vi "Configure TV Trig HDTV Format.vi"(8 "error in (no error)":errorcluster {"code" format="%.0x"}, 10 "HDTV Format (1080I50)":i32(slide), 11 "VISA Resource Name":refnum<visa-resource-name>) -> (0 "error out":errorcluster {"code" format="%.0x"}, 3 "VISA Resource Name Out":refnum<visa-resource-name>)   [LabVIEW 2010, in "Tektronix TDS 3000 Series.lvlib"]
doc: "This VI configures the HDTV settings for the HDTV TV triggering.\n\nNotes:\n\n(1) This VI is effective only if TV Trigger Signal Format in Configure TV Trigger Source is selected as HDTV"
uses:
  <instrlib>/Tektronix TDS 3000 Series/Tektronix TDS 3000 Series.lvlib
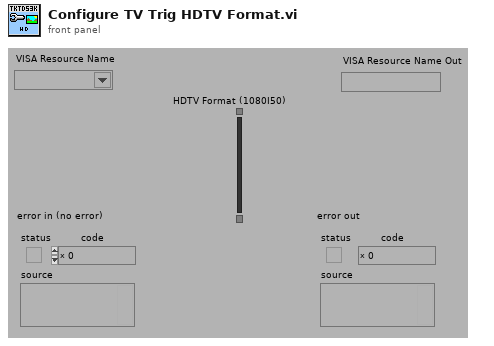
[diagram p1: front panel]
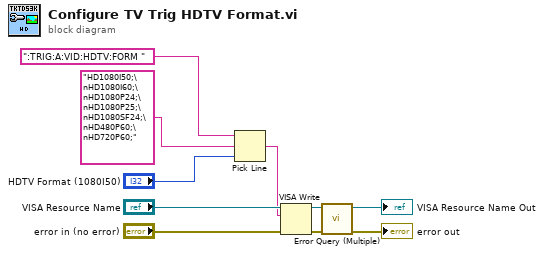
[diagram p0: block diagram]
diagram:
  n1 = Pick Line(string ("")=":TRIG:A:VID:HDTV:FORM " ("format string"), multi-line string="HD1080I50;\nHD1080I60;\nHD1080P24;\nHD1080P25;\nHD1080SF24;\nHD480P60;\nHD720P60;", line index="HDTV Format (1080I50)") -> (output string=w7:string)
  n2 = VISA Write(VISA resource name="VISA Resource Name", write buffer=w7, error in (no error)="error in (no error)") -> (VISA resource name out=w4:refnum<visa-resource-name>, error out=w3:errorcluster)  [unwired: 1 out]
  n3 = call <instrlib>:"Error Query (Multiple).vi"("error in (no error)"=w3, "VISA Resource Name"=w4) -> ("error out"=→"error out":errorcluster, "VISA Resource Name Out"=→"VISA Resource Name Out":refnum<visa-resource-name>)  [unwired: 6 in, 2 out]
